vi "Configure.vi"(8 "error in (no error)":errorcluster, 10 "Configuration":refnum<class "Column Configuration.lvclass">, 11 "Basic Column Factory in":refnum<class "Basic Column Factory.lvclass">) -> (0 "error out":errorcluster, 3 "Basic Column Factory out":refnum<class "Basic Column Factory.lvclass">)   [LabVIEW 2020, in "Basic Columns.lvlib" / "Basic Column Factory.lvclass"]
uses:
  Basic Column Factory.lvclass
  Column Interface/Column Configuration Interface Class/Column Configuration.lvclass
  Basic Column Factory.lvclass/Basic Column Factory.ctl
  Basic Columns/Basic Column Configuration/Basic Column Configuration.lvclass
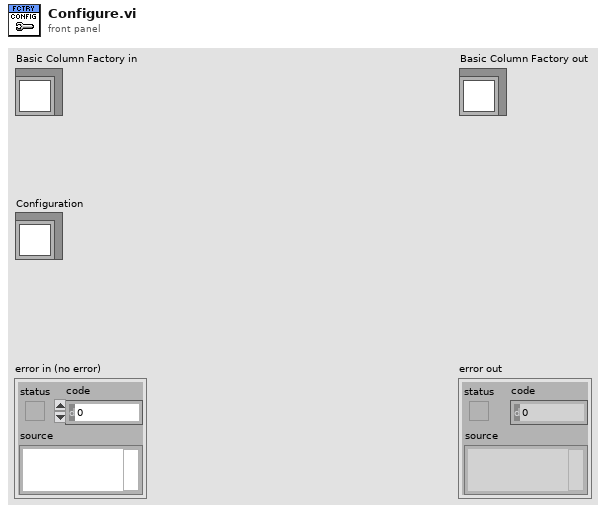
[diagram p1: front panel]
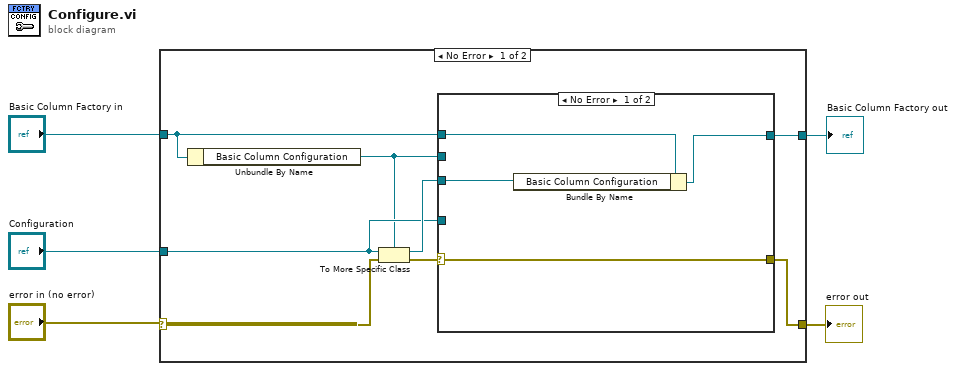
[diagram p0: block diagram]
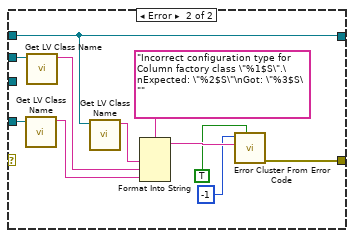
[diagram p2: hidden frame]
diagram:
  n1 = case shown="No Error" "error in (no error)" {
    selector: "error in (no error)" -> [w13 w30]
    tunnel: [w11 w30] -> w2
    tunnel: "Basic Column Factory in" -> [w9 w29]
    tunnel: "Configuration" -> [w7 _]
    tunnel: [w8 w29] -> w1
    frame No Error {
      n2 = Unbundle By Name(w9) -> ("Basic Column Configuration"=w6:refnum<class "Basic Column Configuration.lvclass">)
      n3 = To More Specific Class(target class=w6, reference=w7, error in=w13) -> (specific class reference=w10:refnum<class "Basic Column Configuration.lvclass">, error out=w12:errorcluster)
      n4 = case shown="No Error" w12 {
        selector: w12 -> [w17 _]
        tunnel: [w17 w18] -> w11
        tunnel: w10 -> [w15 _]
        tunnel: w9 -> [w16 w26]
        tunnel: [w14 w26] -> w8
        tunnel: w7 -> [_ w25]
        tunnel: w6 -> [_ w27]
        frame No Error {
          n5 = Bundle By Name(cluster=w16, "Basic Column Configuration"=w15) -> (w14:refnum<class "Basic Column Factory.lvclass">)
        }
        frame Error {
          n6 = call <vilib>:"Get LV Class Name.vi"("object"=w25) -> ("class name"=w22:string)  [unwired: 9 in, 1 out]
          n7 = call <vilib>:"Get LV Class Name.vi"("object"=w27) -> ("class name"=w23:string)  [unwired: 9 in, 1 out]
          n8 = call <vilib>:"Get LV Class Name.vi"("object"=w26) -> ("class name"=w24:string)  [unwired: 9 in, 1 out]
          n9 = Format Into String(format string="Incorrect configuration type for Column factory class \"%1$S\".\nExpected: \"%2$S\"\nGot: \"%3$S\"", w24, w23, w22) -> (resulting string=w21:string)  [unwired: 2 in, 1 out]
          n10 = call <vilib>:"Error Cluster From Error Code.vi"("show call chain? (False)"=TRUE, "error message (\"\")"=w21, "error code (0)"=-1) -> ("error out"=w18:errorcluster)  [unwired: 6 in]
        }
      }
    }
    frame Error {
    }
  }
  "error out" <- w2
  "Basic Column Factory out" <- w1
